vi "closeHandler.vi"(8 "error in (no error)":errorcluster, 11 "Handler.UserEvent in":refnum<class "Handler.UserEvent.lvclass">) -> (0 "error out":errorcluster, 3 "Handler.UserEvent out":refnum<class "Handler.UserEvent.lvclass">)   [LabVIEW 2017, in "Error Log.lvlib" / "Handler.UserEvent.lvclass"]
uses:
  Handler.UserEvent.lvclass
  Handler/Handler.lvclass
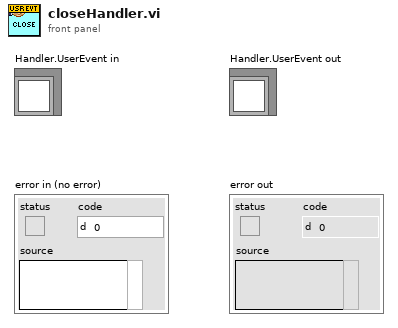
[diagram p1: front panel]
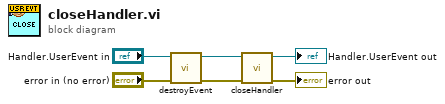
[diagram p0: block diagram]
diagram:
  n1 = call-dynamic "destroyEvent.vi"("error in (no error)"="error in (no error)", "Handler.UserEvent in"="Handler.UserEvent in") -> ("error out"=w1:errorcluster, "Handler.UserEvent out"=w3:refnum<class "Handler.UserEvent.lvclass">)  [unwired: 8 in]
  n2 = call-parent "closeHandler.vi"("error in (no error)"=w1, "Handler in"=w3) -> ("error out"=→"error out":errorcluster, "Handler out"=→"Handler.UserEvent out":refnum<class "Handler.UserEvent.lvclass">)  [unwired: 8 in]
